vi "Read Bypass_.vi"(8 "error in (no error)":errorcluster, 11 "Change Denuded Bypass State in":refnum<class "Change Denuded Bypass State.lvclass">) -> (0 "error out":errorcluster, 2 "Bypass?":bool, 3 "Change Denuded Bypass State out":refnum<class "Change Denuded Bypass State.lvclass">)   [LabVIEW 2014, in "ePAS Library.lvlib" / "Change Denuded Bypass State.lvclass"]
uses:
  Change Denuded Bypass State.lvclass
  Change Denuded Bypass State.lvclass/Change Denuded Bypass State.ctl
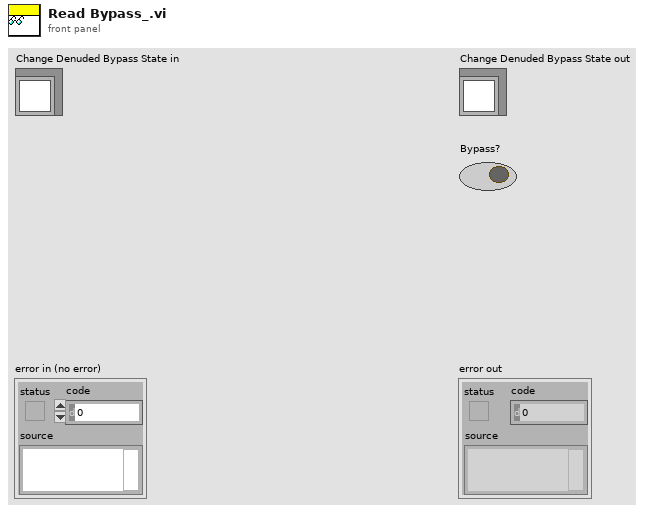
[diagram p1: front panel]
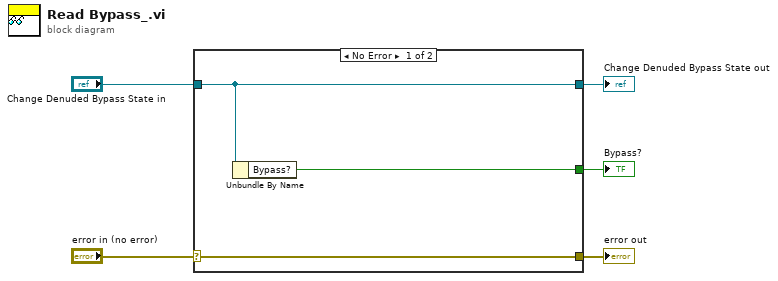
[diagram p0: block diagram]
diagram:
  n1 = case shown="No Error" "error in (no error)" {
    selector: "error in (no error)" -> [w8 w9]
    tunnel: [w8 w9] -> w4
    tunnel: [w7 w10] -> w2
    tunnel: "Change Denuded Bypass State in" -> [w7 w10]
    tunnel: [w6 _] -> w1
    frame No Error {
      n2 = Unbundle By Name(w7) -> ("Bypass?"=w6:bool)
    }
    frame Error {
    }
  }
  "error out" <- w4
  "Change Denuded Bypass State out" <- w2
  "Bypass?" <- w1
